vi "Read Boolean Value.vi"(8 "error in (no error)":errorcluster, 11 "abs_Set_Boolean in":refnum<class "abs_Set_Boolean.lvclass">) -> (0 "error out":errorcluster, 2 "Boolean Value":bool, 3 "abs_Set_Boolean out":refnum<class "abs_Set_Boolean.lvclass">)   [LabVIEW 2021, in "BT.lvlib" / "abs_Set_Boolean.lvclass"]
uses:
  abs_Set_Boolean.lvclass
  abs_Set_Boolean.lvclass/abs_Set_Boolean.ctl
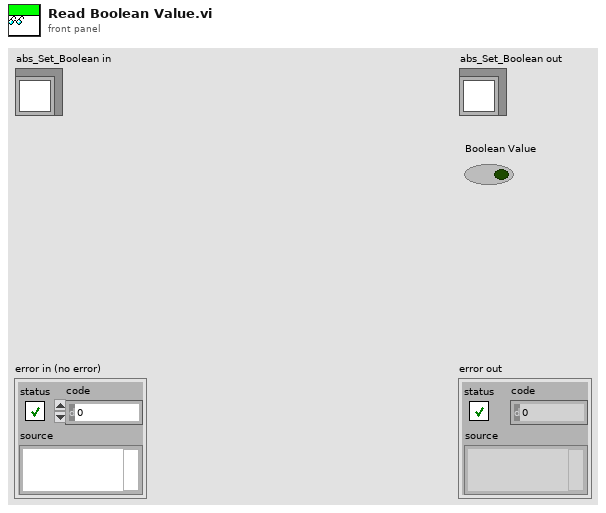
[diagram p1: front panel]
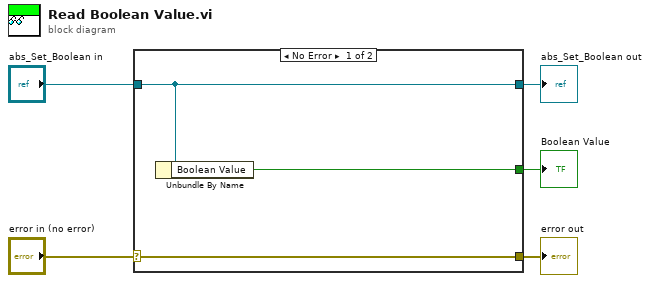
[diagram p0: block diagram]
diagram:
  n1 = case shown="No Error" "error in (no error)" {
    selector: "error in (no error)" -> [w8 w9]
    tunnel: [w8 w9] -> w4
    tunnel: [w7 w10] -> w2
    tunnel: "abs_Set_Boolean in" -> [w7 w10]
    tunnel: [w6 _] -> w1
    frame No Error {
      n2 = Unbundle By Name(w7) -> ("Boolean Value"=w6:bool)
    }
    frame Error {
    }
  }
  "error out" <- w4
  "abs_Set_Boolean out" <- w2
  "Boolean Value" <- w1
